vi "Check Status.vi"(0 "VISA resource name":refnum<visa-resource-name>, 11 "error in (no error)":errorcluster) -> (4 "VISA resource name out":refnum<visa-resource-name>, 15 "error out":errorcluster)   [LabVIEW 2016, in "Fluke 5XXX Series Multicalibrators.lvlib"]
doc: "This VI reads the Standard Event Register and checks it for error. When Error occured, use Error Query VI to describe error type."
uses:
  Fluke 5XXX Series Multicalibrators.lvlib
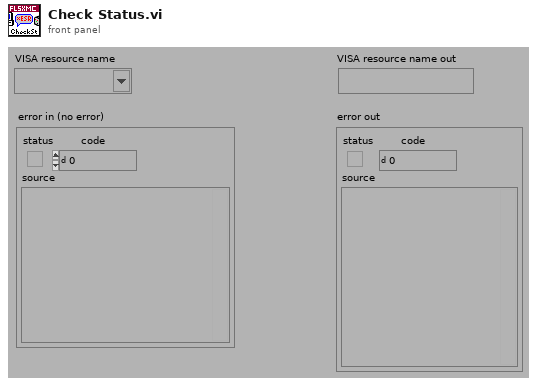
[diagram p1: front panel]
types:
  T1 = cluster{"Status":bool, "Code":i32, "Source (VI Name)":string}
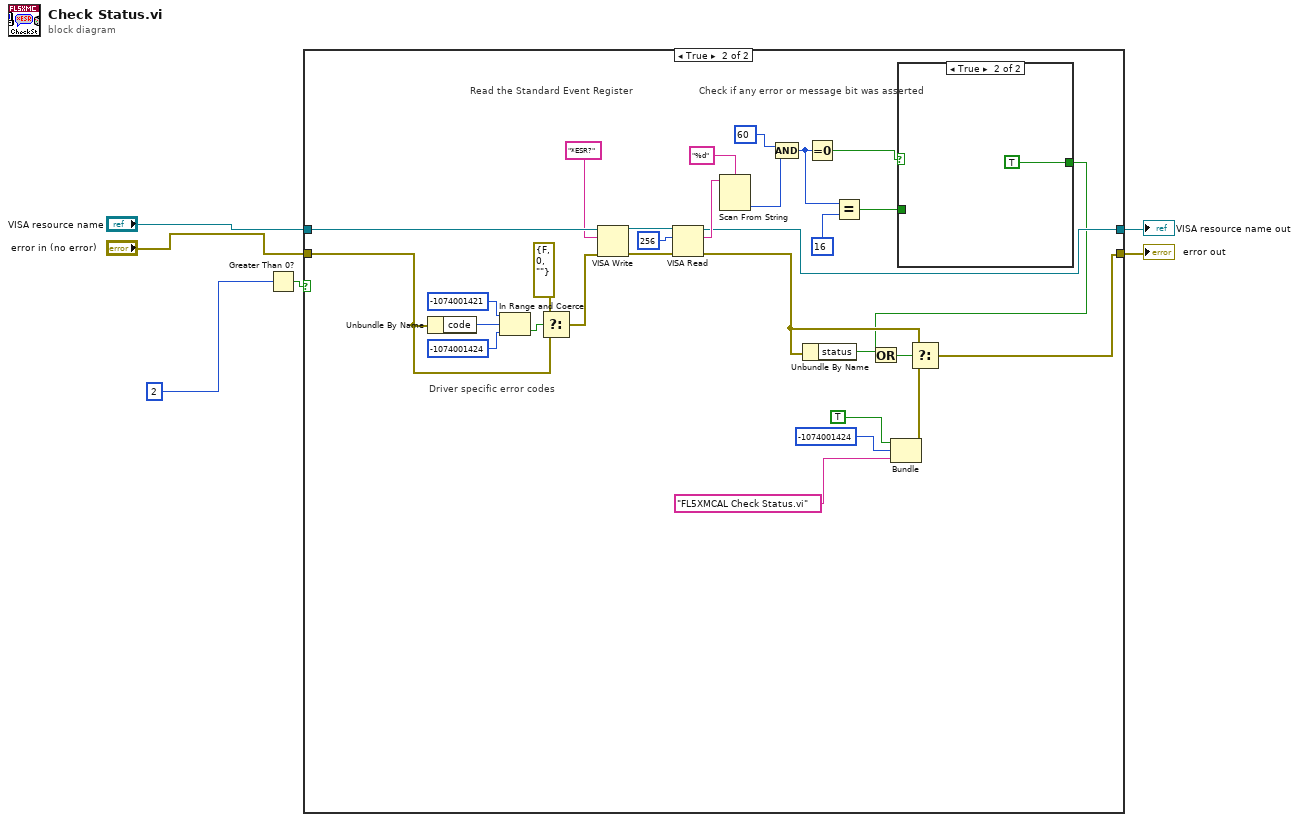
[diagram p0: block diagram]
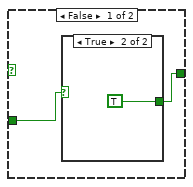
[diagram p3: hidden frame]
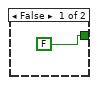
[diagram p4: hidden frame]
diagram:
  n1 = Greater Than 0?(x=2) -> (x > 0?=w4:bool)
  n2 = case shown="True" w4 {
    tunnel: "error in (no error)" -> [w8 w15]
    tunnel: "VISA resource name" -> [w7 w38]
    tunnel: [w7 w23] -> w6
    tunnel: [w8 w21] -> w5
    frame False {
    }
    frame True {
      # "Driver specific error codes"
      # "Check if any error or message bit was asserted"
      # "Read the Standard Event Register"
      n3 = Unbundle By Name(w15) -> ("code"=w18:i32)
      n4 = In Range and Coerce(upper limit=-1074001421, x=w18, lower limit=-1074001424) -> (In Range?=w19:bool)  [unwired: 1 out]
      n5 = Select(t=errorcluster {"status"=FALSE, "code"=0, "source"=""} ("error out"), s=w19, f=w15) -> (s? t:f=w14:errorcluster)
      n6 = VISA Write(VISA resource name=w38, write buffer="*ESR?", error in (no error)=w14) -> (VISA resource name out=w35:refnum<visa-resource-name>, error out=w34:errorcluster)  [unwired: 1 out]
      n7 = VISA Read(VISA resource name=w35, byte count=u32 256 ("byte count (0)"), error in (no error)=w34) -> (VISA resource name out=w23:refnum<visa-resource-name>, read buffer=w32:string, error out=w22:errorcluster)  [unwired: 1 out]
      n8 = Scan From String(format string="%d", input string=w32) -> (output 1=w31:i32)  [unwired: 3 in, 3 out]
      n9 = Compound Arithmetic op=AND(60 ("status"), w31) -> (w11:i32)
      n10 = Unbundle By Name(w22) -> ("status"=w27:bool)
      n11 = Equal To 0?(x=w11) -> (x = 0?=w13:bool)
      n12 = Equal?(x=w11, y=16 ("status")) -> (x = y?=w10:bool)
      n13 = Bundle("Status"=TRUE, "Code"=-1074001424, "Source (VI Name)"="FL5XMCAL Check Status.vi") -> (w26:T1)  [unwired: 1 in]
      n14 = case shown="True" w13 {
        tunnel: [w40 TRUE] -> w12
        tunnel: w10 -> [w39 _]
        frame False {
          n15 = case shown="True" w39 {
            tunnel: [FALSE TRUE] -> w40
            frame False {
            }
            frame True {
            }
          }
        }
        frame True {
        }
      }
      n16 = Or(x=w27, y=w12) -> (x .or. y?=w28:bool)
      n17 = Select(t=w22, s=w28, f=w26) -> (s? t:f=w21:T1)
    }
  }
  "error out" <- w5
  "VISA resource name out" <- w6
